vi "Write number_of_tactics.vi"(8 "error in (no error)":errorcluster, 10 "number_of_tactics":dbl=3.0, 11 "PassObserverRole in":refnum<class "PassObserverRole.lvclass">) -> (0 "error out":errorcluster, 3 "PassObserverRole out":refnum<class "PassObserverRole.lvclass">)   [LabVIEW 2023, in "PassObserverRole.lvclass"]
uses:
  PassObserverRole.lvclass
  PassObserverRole.lvclass/PassObserverRole.ctl
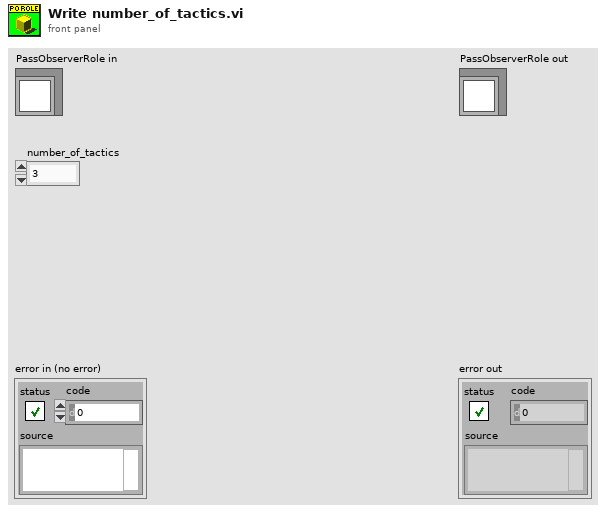
[diagram p1: front panel]
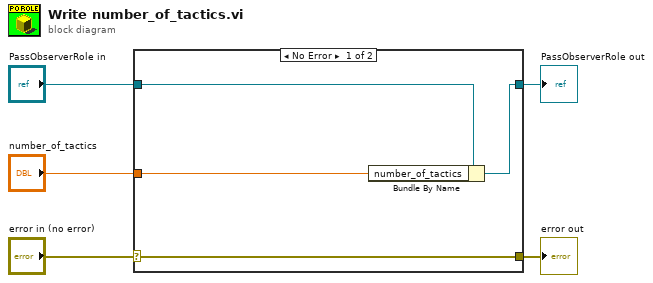
[diagram p0: block diagram]
diagram:
  n1 = case shown="No Error" "error in (no error)" {
    selector: "error in (no error)" -> [w9 w10]
    tunnel: [w9 w10] -> w4
    tunnel: [w7 w11] -> w2
    tunnel: "PassObserverRole in" -> [w8 w11]
    tunnel: "number_of_tactics" -> [w6 _]
    frame No Error {
      n2 = Bundle By Name(cluster=w8, "number_of_tactics"=w6) -> (w7:refnum<class "PassObserverRole.lvclass">)
    }
    frame Error {
    }
  }
  "error out" <- w4
  "PassObserverRole out" <- w2
